vi "JSON String to Step.vi"(8 "error in (no error)":errorcluster, 10 "JSON String":string, 11 "Base Step in":refnum<class "Base Step.lvclass">) -> (0 "error out":errorcluster, 3 "Base Step out":refnum<class "Base Step.lvclass">)   [LabVIEW 2024, in "Ramses Sequencer.lvlib" / "Base Step.lvclass"]
uses:
  Base Step.lvclass
  Typedefs/Step State.ctl
  <vilib>/Utility/Data Type/Type Definitions/Data Type.ctl
  ea568c66-cc00-4458-a224-cee80663da2d.vi
  <vilib>/JDP Science/JSONtext/LVClass Serializer/JSONtext LVClass Serializer.lvclass
  <vilib>/Utility/Data Type/NI_Data Type.lvlib
  <vilib>/JDP Science/JSONtext/JSONtext.lvlib
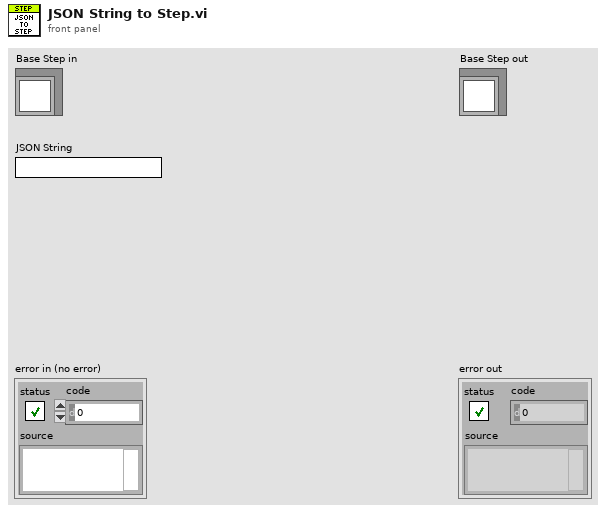
[diagram p1: front panel]
types:
  T1 = typedef "Ramses Sequencer.lvlib/Base Step.lvclass/Step State.ctl" = cluster{"Result":string, "Status":string, "Enabled":bool, "Upper":string, "Target":string, "Lower":string, "Value":string}
  T2 = typedef "NI_Data Type.lvlib/Data Type.ctl" = enum8{"Invalid Type", "Void", "I8", "I16", "I32", "I64", "U8", "U16", "U32", "U64", "Single Float", "Double Float", "Extended Float", "Single Complex", "Double Complex", "Extended Complex", "Enum U8", "Enum U16", "Enum U32", "Enum U64", "Single Float With Unit", "Double Float With Unit", "Extended Float With Unit", "Single Complex with Unit", "Double Complex with Unit", "Extended Complex with Unit", "Boolean", "String", "Path", "Picture", "Tag", "Array", "Cluster", "Variant", "LV Variant", "Waveform", "Timestamp", "Digital Waveform", "Digital Data", "ExpressData", "Refnum", "External Data", "VI", "Poly VI", "LabVIEW Class Instance", "Fixed Point", "Set Collection", "Map Collection"}
  T3 = cluster{"Class Name":string, "Name":string, "Step State":T1, "Properties":cluster{string, "type":T2, "<JSON>":string}[]}
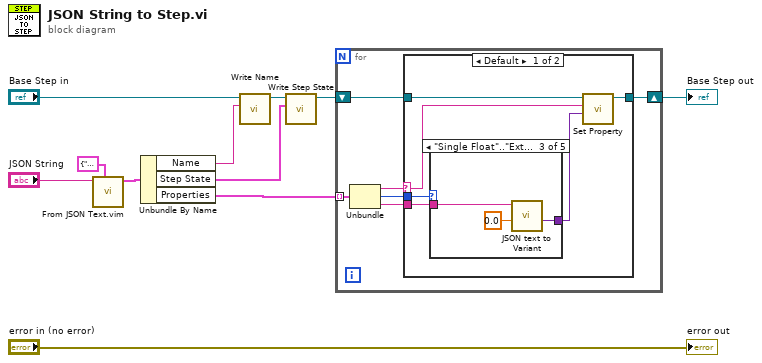
[diagram p0: block diagram]
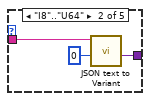
[diagram p3: hidden frame]
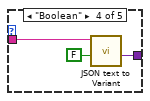
[diagram p4: hidden frame]
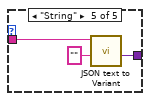
[diagram p5: hidden frame]
diagram:
  n1 = call "From JSON Text.vim"("Data Type and Default Value"=T3 {"Class Name"="", "Name"="", "Step State"={"Result"="", "Status"="", "Enabled"=FALSE, "Upper"="", "Target"="", "Lower"="", "Value"=""}, "Properties"=[]} ("cluster"), "JSON"="JSON String") -> ("Data out"=w9:T3)  [unwired: 8 in, 1 out]
  n2 = Unbundle By Name(w9) -> ("Name"=w5:string, "Step State"=w2:T1, "Properties"=w7:cluster{string, "type":T2, "<JSON>":string}[])
  n3 = call-dynamic "Write Name.vi"("Name"=w5, "Base Step in"="Base Step in") -> ("Base Step out"=w4:refnum<class "Base Step.lvclass">)  [unwired: 8 in, 1 out]
  n4 = call "Write Step State.vi"("Step State"=w2, "Base Step in"=w4) -> ("Base Step out"=w3:refnum<class "Base Step.lvclass">)  [unwired: 8 in, 1 out]
  n5 = for {
    tunnel: w7 -> [w17] mode=indexing
    shift-right: [w15] -> w6
    shift-left: w3 -> [w16]
    n6 = Unbundle(w17) -> (w14:string, "type"=w13:T2, "<JSON>"=w12:string)
    n7 = case shown="Default" w14 {
      selector: w14 -> [w21 _]
      tunnel: w16 -> [w23 w36]
      tunnel: [w22 w36] -> w15
      tunnel: w13 -> [w20 _]
      tunnel: w12 -> [w19 _]
      frame Default {
        n8 = case shown="\"Single Float\"..\"Extended Float\"" w20 {
          tunnel: w19 -> [_ w26 w29 w32 w35]
          tunnel: [_ w24 w27 w30 w33] -> w18
          frame Default {
          }
          frame "I8".."U64" {
            n9 = call <vilib>:"JSON text to Variant.vi"("Data Type"=0, "JSON"=w26) -> ("Variant out"=w24:variant)  [unwired: 8 in, 1 out]
          }
          frame "Single Float".."Extended Float" {
            n10 = call <vilib>:"JSON text to Variant.vi"("Data Type"=0.0, "JSON"=w29) -> ("Variant out"=w27:variant)  [unwired: 8 in, 1 out]
          }
          frame "Boolean" {
            n11 = call <vilib>:"JSON text to Variant.vi"("Data Type"=FALSE, "JSON"=w32) -> ("Variant out"=w30:variant)  [unwired: 8 in, 1 out]
          }
          frame "String" {
            n12 = call <vilib>:"JSON text to Variant.vi"("Data Type"="", "JSON"=w35) -> ("Variant out"=w33:variant)  [unwired: 8 in, 1 out]
          }
        }
        n13 = call "Set Property.vi"("Data"=w18, "Key"=w21, "Base Step in"=w23) -> ("Base Step out"=w22:refnum<class "Base Step.lvclass">)  [unwired: 7 in, 1 out]
      }
      frame "Step State" {
      }
    }
  }
  "Base Step out" <- w6
  "error out" <- "error in (no error)"
